vi "Inputs.vi"(8 "error in (no error)":errorcluster, 11 "RGetInputList in":refnum<class "RGetInputList.lvclass">) -> (0 "error out":errorcluster, 2 "Inputs":T1[](array[typedef]), 3 "RGetInputList out":refnum<class "RGetInputList.lvclass">)   [LabVIEW 2020, in "obs-websocket.lvlib" / "RGetInputList.lvclass"]
uses:
  RGetInputList.lvclass
  RGetInputList.lvclass/RGetInputList.ctl
  Input.ctl
  obs-websocket.lvlib
  Input Settings.ctl
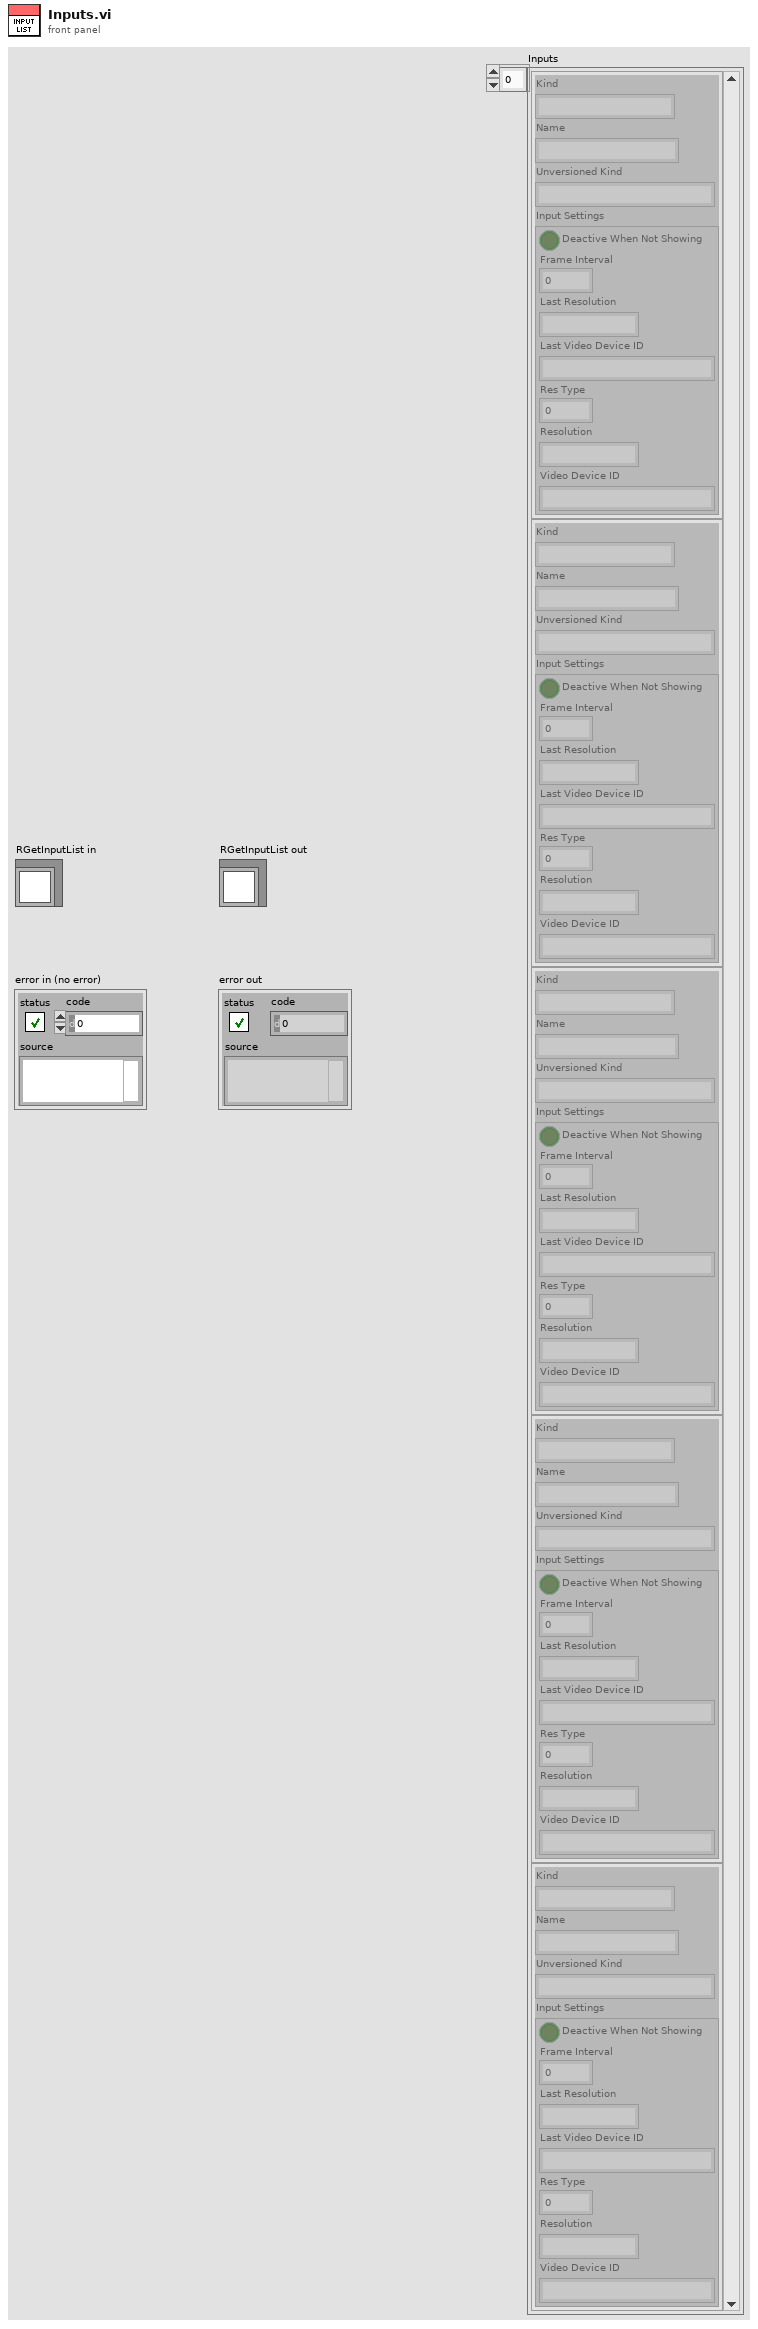
[diagram p1: front panel]
types:
  T1 = typedef "obs-websocket.lvlib/Input.ctl" = cluster{"Kind":string, "Name":string, "Unversioned Kind":string, "Input Settings":T2}
  T2 = typedef "obs-websocket.lvlib/Input Settings.ctl" = cluster{"Deactive When Not Showing":bool, "Frame Interval":i32, "Last Resolution":string, "Last Video Device ID":string, "Res Type":i32, "Resolution":string, "Video Device ID":string}
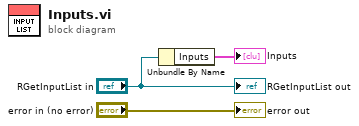
[diagram p0: block diagram]
diagram:
  n1 = Unbundle By Name("RGetInputList in") -> ("Inputs"=→"Inputs":T1[])
  "error out" <- "error in (no error)"
  "RGetInputList out" <- "RGetInputList in"
